vi "Ausgangswinkel.vi"(1 "Hauswinkel":dbl, 2 "Einfallswinkel":dbl) -> (0 "Stellwinkel":dbl)   [LabVIEW 2013]
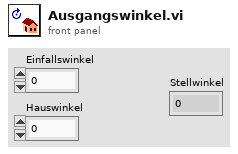
[diagram p1: front panel]
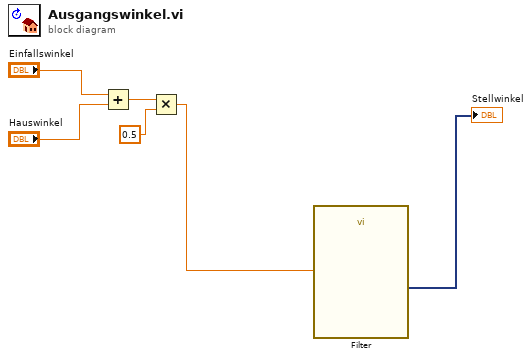
[diagram p0: block diagram]
diagram:
  n1 = Add(x="Einfallswinkel", y="Hauswinkel") -> (x+y=w4:dbl)
  n2 = Multiply(x=w4, y=0.5) -> (x*y=w2:dbl)
  n3 = call "Filter"("Signal"=w2) -> ("Filtered Signal"=→"Stellwinkel":dynamicdata)  [unwired: 9 in, 1 out]
